vi "PIDController_AdvExecute.vi"(4 "Reset":bool, 5 "PID Error Tolerance":T2={"PositionTolerance"=0.001, "VelocityTolerance"=9.9e+30}, 6 "Auto":bool=TRUE, 7 "Adv PID Limits":T1={"MaxInput"=0.0, "MinInput"=0.0, "Continuous"=FALSE, "MaxOutput"=9.9e+32, "MinOutput"=-9.9e+32}, 8 "FF-FeedForward":dbl, 9 "SP-SetPoint":dbl, 10 "PV-Measurement":dbl, 11 "Adv PID Tuning":T3={"Kf"=0.0, "Kp"=0.0, "Ki"=0.0, "Kd"=0.0, "MaximumIntegral"=9.9e+30, "MinimumIntegral"=-9.9e+30, "Filter Derivative"=FALSE}) -> (0 "AtSetpoint":bool, 1 "CO-ControlOutput":dbl, 3 "out PID_CONTROLLER":T4={"Kp"=0.0, "Ki"=0.0, "Kd"=0.0, "Period"=0.0, "Max_Integral"=0.0, "Min_Integral"=0.0, "Max_Input"=0.0, "Min_Input"=0.0, "Continuous"=FALSE, "PositionError"=0.0, "VelocityError"=0.0, "PrevError"=0.0, "TotalError"=0.0, "PositionTolerance"=0.0, "VelocityTolerance"=0.0, "SetPoint"=0.0, "Kf"=0.0, "Prev_Deriv"=0.0, "Prev_Deriv 2"=0.0, "DerivativeFilter"=FALSE, "Min_Output"=-9.99e+35, "Max_Output"=9.9e+35, "Prev_F_P"=0.0, "Prev_F_P_2"=0.0, "AntiWindupActive"=FALSE} {"Prev_F_P_2" format="%16_6e"; "Prev_F_P" format="%16_6e"; "Max_Output" format="%16_6e"; "Min_Output" format="%16_6e"; "Prev_Deriv 2" format="%16_6e"; "Prev_Deriv" format="%16_6e"; "Kf" format="%16_6e"; "SetPoint" format="%16_6e"; "VelocityTolerance" format="%16_6e"; "PositionTolerance" format="%16_6e"; "TotalError" format="%16_6e"; "PrevError" format="%16_6e"; "VelocityError" format="%16_6e"; "PositionError" format="%16_6e"; "Min_Input" format="%16_6e"; "Max_Input" format="%16_6e"; "Min_Integral" format="%16_6e"; "Max_Integral" format="%16_6e"; "Period" format="%16_6e"; "Kd" format="%16_6e"; "Ki" format="%16_6e"; "Kp" format="%16_6e"})   [LabVIEW 2019, in "Trajectory_Library.lvlib"]
doc: "Convience, single call, LabVIEW function. Creates and calculates the \"advanced\" PID controller. Call this routine periodically to calculate the newest output for the provided inputs. \n\nSee the \"PID Adv Calculate\" VI documentation for additional details on the \"advanced PID\"\n \nInputs:\n - PID Error Tolerance -- Tolerances for determining \"At Setpoint\", contains:\n - Position Tolerance -- (Default: 0.001)\n - Velocity Tolerance -- (Default: 9.9E+30)\n - Adv PID Limits -- Cluster containing:\n - MaxInput -- (Default: 0)\n - MinInput -- (Default: 0)\n - Continous -- When True indicates that the input is continuous. (Default: False)\n - MaxOutput -- The largest allowed value for the control output (CO) \n - MinOutput -- The smallest allowed value for the control output (CO)\n - PID Tuning -- PID Tuning parameters containing:\n - Kf -- The feedforward gain coefficient.\n - Kp -- The proportional coefficient.\n - Ki -- The integral coefficient.\n - Kd -- The derivative coefficient.\n - Maximum Integral -- The maximum value of the integrator.\n - Minimum Integral -- The minimum value of the integrator.\n - Filter Derivative -- Use derivative filtering when True.\n - PV-measurement -- The current measurement of the process variable. (PV)\n - SP-setpoint -- The new setpoint of the controller. (SP)\n - FF-Feedforward -- The feedforward value. \n - Auto -- Use the PID calculate when this is True\n - Reset -- When True, causes the PID to be reset. (Default: False)\n\nOutputs:\n - PID_Controller -- Updated PID_Controller data cluster\n - CO-ControlOutput -- Controller output (CO) \n - AtSetpoint -- True when PV is within the specified tolerances of the SP."
uses:
  Trajectory_Library.lvlib
  PID_CONTROLLER.ctl
  PID_ERROR_TOLERANCE.ctl
  PID_ADV_LIMITS.ctl
  PID_ADV_TUNING.ctl
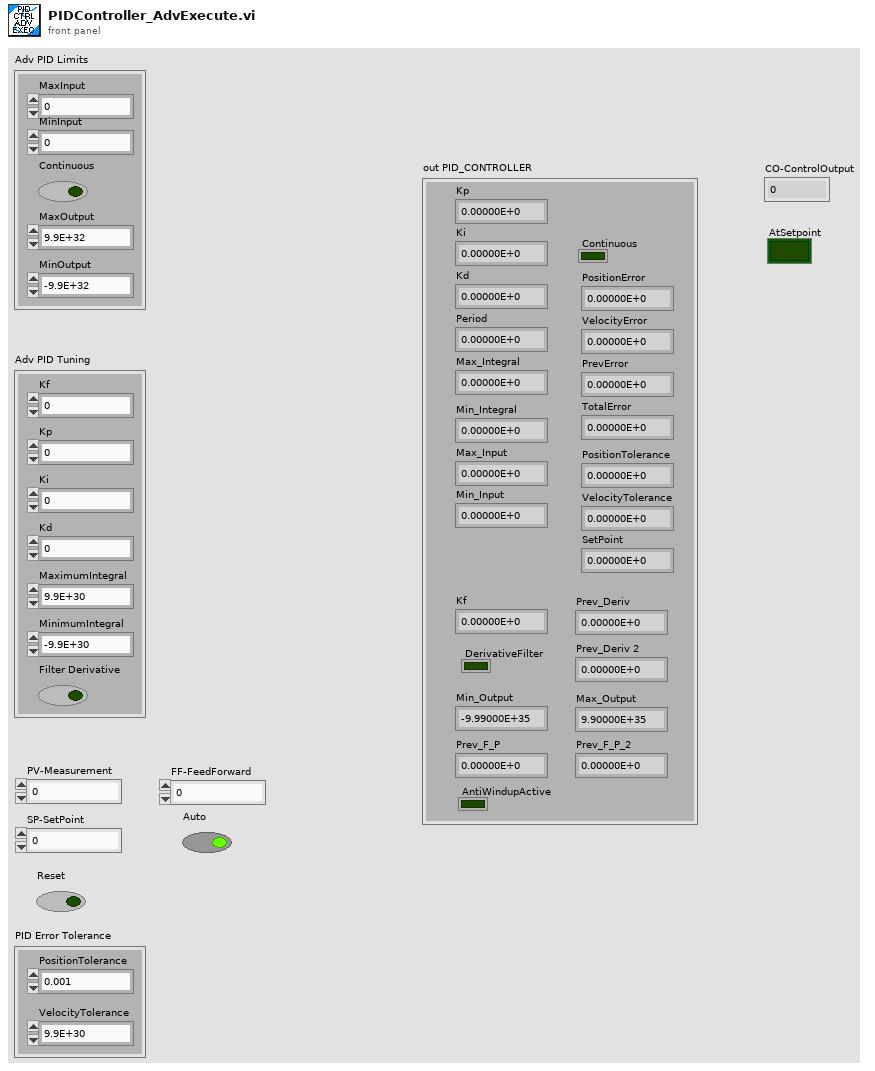
[diagram p1: front panel]
types:
  T1 = typedef "Trajectory_Library.lvlib/PID_ADV_LIMITS.ctl" = cluster{"MaxInput":dbl, "MinInput":dbl, "Continuous":bool, "MaxOutput":dbl, "MinOutput":dbl}
  T2 = typedef "Trajectory_Library.lvlib/PID_ERROR_TOLERANCE.ctl" = cluster{"PositionTolerance":dbl, "VelocityTolerance":dbl}
  T3 = typedef "Trajectory_Library.lvlib/PID_ADV_TUNING.ctl" = cluster{"Kf":dbl, "Kp":dbl, "Ki":dbl, "Kd":dbl, "MaximumIntegral":dbl, "MinimumIntegral":dbl, "Filter Derivative":bool}
  T4 = typedef "Trajectory_Library.lvlib/PID_CONTROLLER.ctl" = cluster{"Kp":dbl, "Ki":dbl, "Kd":dbl, "Period":dbl, "Max_Integral":dbl, "Min_Integral":dbl, "Max_Input":dbl, "Min_Input":dbl, "Continuous":bool, "PositionError":dbl, "VelocityError":dbl, "PrevError":dbl, "TotalError":dbl, "PositionTolerance":dbl, "VelocityTolerance":dbl, "SetPoint":dbl, "Kf":dbl, "Prev_Deriv":dbl, "Prev_Deriv 2":dbl, "DerivativeFilter":bool, "Min_Output":dbl, "Max_Output":dbl, "Prev_F_P":dbl, "Prev_F_P_2":dbl, "AntiWindupActive":bool}
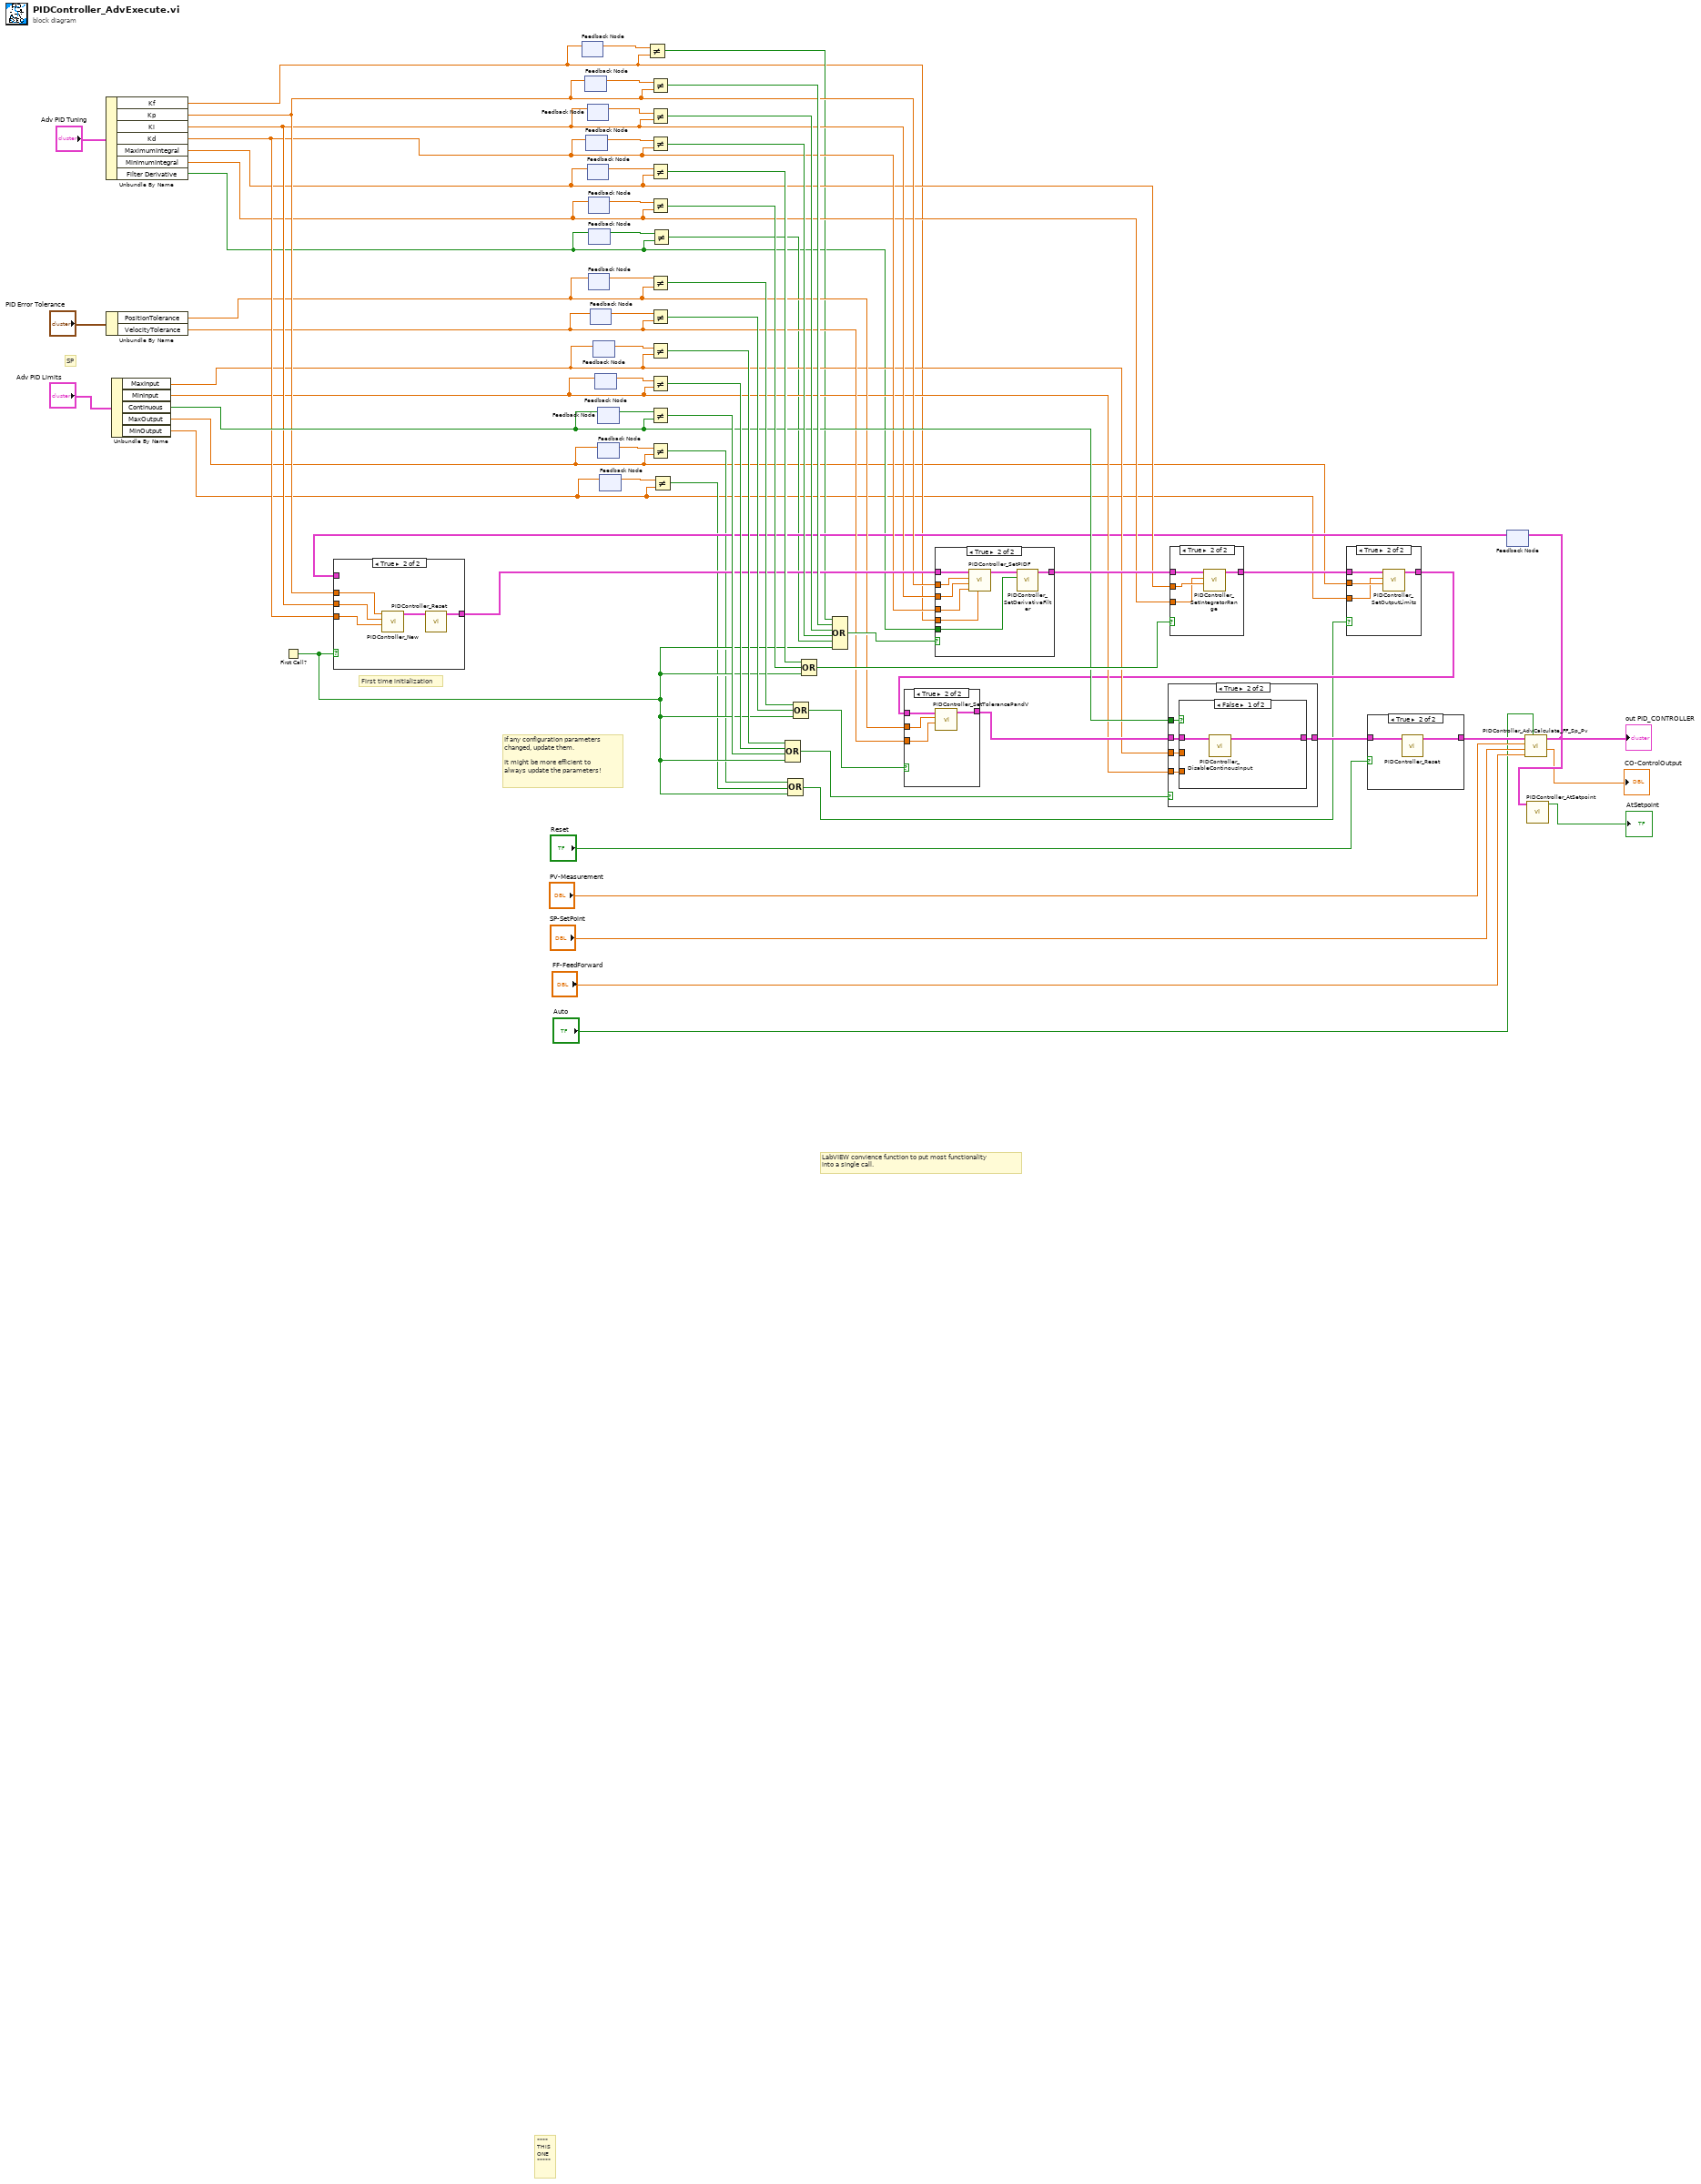
[diagram p0: block diagram]
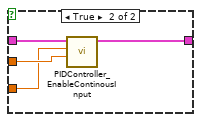
[diagram p6: hidden frame]
diagram:
  # "First time initialization"
  # "If any configuration parameters \nchanged, update them.\n\nIt might be more efficient to\nalways update the parameters!"
  # "SP"
  # "LabVIEW convience function to put most functionality\ninto a single call."
  # "****\nTHIS\nONE\n*****"
  n1 = Unbundle By Name("Adv PID Tuning") -> ("Kf"=w14:dbl, "Kp"=w42:dbl, "Ki"=w41:dbl, "Kd"=w40:dbl, "MaximumIntegral"=w39:dbl, "MinimumIntegral"=w38:dbl, "Filter Derivative"=w11:bool)
  n2 = Unbundle By Name("PID Error Tolerance") -> ("PositionTolerance"=w37:dbl, "VelocityTolerance"=w36:dbl)
  n3 = Unbundle By Name("Adv PID Limits") -> ("MaxInput"=w35:dbl, "MinInput"=w34:dbl, "Continuous"=w44:bool, "MaxOutput"=w2:dbl, "MinOutput"=w1:dbl)
  n4 = First Call?() -> (First Call?: T/F=w8:bool)
  n5 = feedback #1() -> (w16:dbl)  [unwired: 1 in]
  n6 = feedback-in #1(w14) -> ()
  n7 = feedback #2() -> (w33:dbl)  [unwired: 1 in]
  n8 = feedback-in #2(w42) -> ()
  n9 = feedback #3() -> (w31:dbl)  [unwired: 1 in]
  n10 = feedback-in #3(w40) -> ()
  n11 = feedback #4() -> (w32:dbl)  [unwired: 1 in]
  n12 = feedback-in #4(w41) -> ()
  n13 = feedback #5() -> (w30:dbl)  [unwired: 1 in]
  n14 = feedback-in #5(w39) -> ()
  n15 = feedback #6() -> (w29:dbl)  [unwired: 1 in]
  n16 = feedback-in #6(w38) -> ()
  n17 = feedback #7() -> (w28:dbl)  [unwired: 1 in]
  n18 = feedback-in #7(w37) -> ()
  n19 = feedback #8() -> (w13:bool)  [unwired: 1 in]
  n20 = feedback-in #8(w11) -> ()
  n21 = feedback #9() -> (w27:dbl)  [unwired: 1 in]
  n22 = feedback-in #9(w36) -> ()
  n23 = feedback #10() -> (w26:dbl)  [unwired: 1 in]
  n24 = feedback-in #10(w35) -> ()
  n25 = feedback #11() -> (w25:dbl)  [unwired: 1 in]
  n26 = feedback-in #11(w34) -> ()
  n27 = feedback-in #12(w44) -> ()
  n28 = feedback #12() -> (w43:bool)  [unwired: 1 in]
  n29 = feedback #13() -> (w6:dbl)  [unwired: 1 in]
  n30 = feedback-in #13(w2) -> ()
  n31 = feedback #14() -> (w5:dbl)  [unwired: 1 in]
  n32 = feedback-in #14(w1) -> ()
  n33 = Not Equal?(x=w16, y=w14) -> (x != y?=w15:bool)
  n34 = Not Equal?(x=w33, y=w42) -> (x != y?=w53:bool)
  n35 = Not Equal?(x=w32, y=w41) -> (x != y?=w54:bool)
  n36 = Not Equal?(x=w31, y=w40) -> (x != y?=w55:bool)
  n37 = Not Equal?(x=w30, y=w39) -> (x != y?=w56:bool)
  n38 = Not Equal?(x=w29, y=w38) -> (x != y?=w57:bool)
  n39 = Not Equal?(x=w28, y=w37) -> (x != y?=w58:bool)
  n40 = Not Equal?(x=w27, y=w36) -> (x != y?=w59:bool)
  n41 = Not Equal?(x=w26, y=w35) -> (x != y?=w60:bool)
  n42 = Not Equal?(x=w25, y=w34) -> (x != y?=w61:bool)
  n43 = Not Equal?(x=w43, y=w44) -> (x != y?=w62:bool)
  n44 = Not Equal?(x=w6, y=w2) -> (x != y?=w4:bool)
  n45 = Not Equal?(x=w13, y=w11) -> (x != y?=w12:bool)
  n46 = Not Equal?(x=w5, y=w1) -> (x != y?=w3:bool)
  n47 = Compound Arithmetic op=OR(w60, w61, w62, w8) -> (w48:bool)
  n48 = Compound Arithmetic op=OR(w4, w3, w8) -> (w7:bool)
  n49 = Compound Arithmetic op=OR(w58, w59, w8) -> (w49:bool)
  n50 = Compound Arithmetic op=OR(w56, w57, w8) -> (w50:bool)
  n51 = Compound Arithmetic op=OR(w15, w53, w54, w55, w12, w8) -> (w52:bool)
  n52 = feedback #15() -> (w24:T4)  [unwired: 1 in]
  n53 = case shown="True" w8 {
    tunnel: w42 -> [_ w71]
    tunnel: w41 -> [_ w70]
    tunnel: w40 -> [_ w69]
    tunnel: [w68 w73] -> w45
    tunnel: w24 -> [w68 _]
    frame False {
    }
    frame True {
      n54 = call "PIDController_New.vi"("Kd"=w69, "Ki"=w70, "Kp"=w71) -> ("PID_CONTROLLER"=w72:T4)  [unwired: 8 in]
      n55 = call "PIDController_Reset.vi"("in PID_CONTROLLER"=w72) -> ("out PID_CONTROLLER"=w73:T4)  [unwired: 10 in]
    }
  }
  n56 = case shown="True" w52 {
    tunnel: w45 -> [w74 w82]
    tunnel: w42 -> [_ w81]
    tunnel: w41 -> [_ w80]
    tunnel: w40 -> [_ w79]
    tunnel: [w74 w77] -> w51
    tunnel: w14 -> [_ w78]
    tunnel: w11 -> [_ w75]
    frame False {
    }
    frame True {
      n57 = call "PIDController_SetPIDF.vi"("Kf"=w78, "Kd"=w79, "Ki"=w80, "Kp"=w81, "in PID_CONTROLLER"=w82) -> ("out PID_CONTROLLER"=w76:T4)  [unwired: 6 in]
      n58 = call "PIDController_SetDerivativeFilter.vi"("DerivativeFilter"=w75, "in PID_CONTROLLER"=w76) -> ("out PID_CONTROLLER"=w77:T4)  [unwired: 9 in]
    }
  }
  n59 = case shown="True" w50 {
    tunnel: w51 -> [w83 w87]
    tunnel: w39 -> [_ w86]
    tunnel: w38 -> [_ w85]
    tunnel: [w83 w84] -> w10
    frame False {
    }
    frame True {
      n60 = call "PIDController_SetIntegratorRange.vi"("MaximumIntegral"=w86, "MinimumIntegral"=w85, "in PID_CONTROLLER"=w87) -> ("out PID_CONTROLLER"=w84:T4)  [unwired: 8 in]
    }
  }
  n61 = case shown="True" w7 {
    tunnel: w10 -> [w88 w92]
    tunnel: [w88 w91] -> w9
    tunnel: w2 -> [_ w90]
    tunnel: w1 -> [_ w89]
    frame False {
    }
    frame True {
      n62 = call "PIDController_SetOutputLimits.vi"("MaxOutput"=w90, "MinOutput"=w89, "in PID_CONTROLLER"=w92) -> ("out PID_CONTROLLER"=w91:T4)  [unwired: 8 in]
    }
  }
  n63 = case shown="True" w49 {
    tunnel: w9 -> [w93 w97]
    tunnel: w37 -> [_ w96]
    tunnel: w36 -> [_ w95]
    tunnel: [w93 w94] -> w47
    frame False {
    }
    frame True {
      n64 = call "PIDController_SetTolerancePandV.vi"("VelocityTolerance"=w95, "PositionTolerance"=w96, "in PID_CONTROLLER"=w97) -> ("out PID_CONTROLLER"=w94:T4)  [unwired: 8 in]
    }
  }
  n65 = case shown="True" w48 {
    tunnel: w35 -> [_ w103]
    tunnel: w34 -> [_ w102]
    tunnel: w47 -> [w98 w101]
    tunnel: w44 -> [_ w100]
    tunnel: [w98 w99] -> w46
    frame False {
    }
    frame True {
      n66 = case shown="False" w100 {
        tunnel: w101 -> [w105 w109]
        tunnel: [w104 w108] -> w99
        tunnel: w103 -> [_ w107]
        tunnel: w102 -> [_ w106]
        frame False {
          n67 = call "PIDController_DisableContinousInput.vi"("in PID_CONTROLLER"=w105) -> ("out PID_CONTROLLER"=w104:T4)  [unwired: 10 in]
        }
        frame True {
          n68 = call "PIDController_EnableContinousInput.vi"("MaxInput"=w107, "MinInput"=w106, "in PID_CONTROLLER"=w109) -> ("out PID_CONTROLLER"=w108:T4)  [unwired: 8 in]
        }
      }
    }
  }
  n69 = case shown="True" "Reset" {
    tunnel: w46 -> [w110 w112]
    tunnel: [w110 w111] -> w21
    frame False {
    }
    frame True {
      n70 = call "PIDController_Reset.vi"("in PID_CONTROLLER"=w112) -> ("out PID_CONTROLLER"=w111:T4)  [unwired: 10 in]
    }
  }
  n71 = call "PIDController_AdvCalculate_FF_Sp_Pv.vi"("Auto"="Auto", "FF"="FF-FeedForward", "SP"="SP-SetPoint", "PV"="PV-Measurement", "in PID_CONTROLLER"=w21) -> ("ControlOutput"=→"CO-ControlOutput":dbl, "out PID_CONTROLLER"=w23:T4)  [unwired: 5 in]
  "out PID_CONTROLLER" <- w23
  n72 = feedback-in #15(w23) -> ()
  n73 = call "PIDController_AtSetpoint.vi"("in PID_CONTROLLER"=w23) -> ("AtSetpoint"=→"AtSetpoint":bool)  [unwired: 10 in]
